vi "enable logging.vi"(6 "call chain index (1)":i32, 7 "vi ref (caller)":refnum<vi>, 8 "error in (no error)":errorcluster, 10 "save pre-launch status (F)":bool, 11 "log file path":path) -> (0 "error out":errorcluster)   [LabVIEW 2024, in "status manager.lvlib"]
uses:
  status manager.lvlib
  <vilib>/Hampel Software Engineering/HSE Logger/LogLevel.ctl
  logger actions.ctl
  <vilib>/Hampel Software Engineering/HSE Logger/Formatter/HSE_v2_Formatter/HSE_v2_Formatter.lvclass
  <vilib>/Hampel Software Engineering/HSE Logger/Handler/FileHandler/FileHandler.lvclass
  <vilib>/Hampel Software Engineering/HSE Logger/hse-logger.lvlib
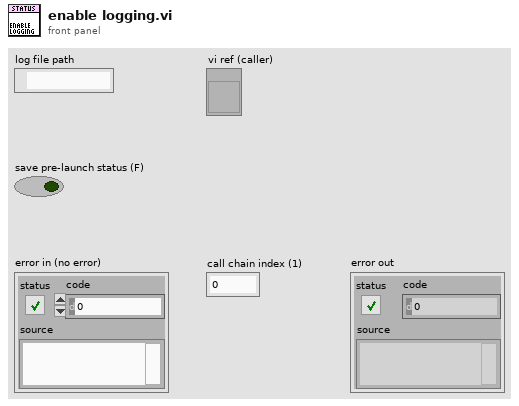
[diagram p1: front panel]
types:
  T1 = typedef "status manager.lvlib/logger actions.ctl" = enum16{"insert", "remove"}
  T2 = typedef "hse-logger.lvlib/LogLevel.ctl" = enum16{"DEBUG", "INFO", "WARNING", "ERROR", "CRITICAL"}
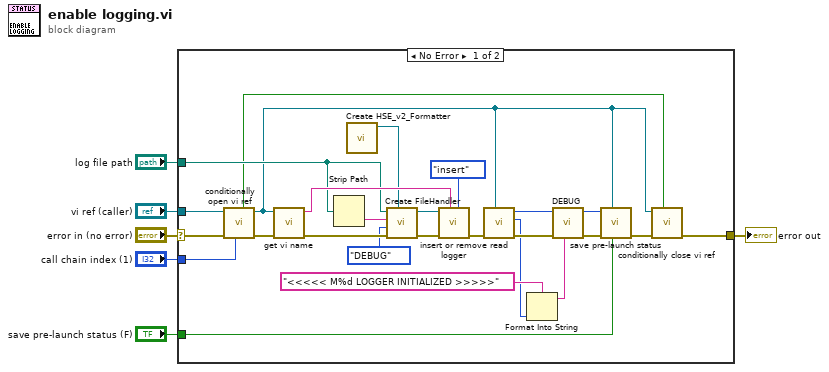
[diagram p0: block diagram]
diagram:
  n1 = case shown="No Error" "error in (no error)" {
    selector: "error in (no error)" -> [w19 w32]
    tunnel: "log file path" -> [w26 _]
    tunnel: "vi ref (caller)" -> [w17 _]
    tunnel: [w22 w32] -> w3
    tunnel: "save pre-launch status (F)" -> [w20 _]
    tunnel: "call chain index (1)" -> [w9 _]
    frame No Error {
      n2 = call "conditionally open vi ref.vi"("call chain index (1)"=w9, "error in (no error)"=w19, "vi ref in"=w17) -> ("error out"=w18:errorcluster, "vi ref out"=w8:refnum<vi>, "new ref?"=w16:bool)  [unwired: 6 in]
      n3 = call "get vi name.vi"("error in (no error)"=w18, "vi ref"=w8) -> ("error out"=w30:errorcluster, "vi name"=w31:string)  [unwired: 8 in]
      n4 = Strip Path(path=w26) -> (name=w25:string)  [unwired: 1 out]
      n5 = call <vilib>:"Create HSE_v2_Formatter.vi"() -> ("HSE_v2_Formatter out"=w27:refnum<class "HSE_v2_Formatter.lvclass">)  [unwired: 10 in, 1 out]
      n6 = call <vilib>:"Create FileHandler.vi"("Formatter.lvclass"=w27, "error in"=w30, "Level"=LogLevel."DEBUG", "Name"=w25, "Filepath"=w26) -> ("error out"=w15:errorcluster, "FileHandler out"=w13:refnum<class "FileHandler.lvclass">)  [unwired: 5 in]
      n7 = call "insert or remove logger.vi"("action"=logger_actions."insert", "handler name"=w31, "error in (no error)"=w15, "handler to insert"=w13) -> ("error out"=w14:errorcluster)  [unwired: 7 in]
      n8 = call "read.vi"("vi ref (caller)"=w8, "error in (no error)"=w14) -> ("error out"=w11:errorcluster, "module id"=w10:i32, "status control id"=w7:i32)  [unwired: 7 in]
      n9 = Format Into String(format string="<<<<< M%d LOGGER INITIALIZED >>>>>", w10) -> (resulting string=w23:string)  [unwired: 2 in, 1 out]
      n10 = call <vilib>:"DEBUG.vi"("Message"=w23, "error in"=w11) -> ("error out"=w29:errorcluster)  [unwired: 9 in]
      n11 = call "save pre-launch status.vi"("save pre-launch status"=w20, "vi ref"=w8, "error in (no error)"=w29, "status control id"=w7) -> ("error out"=w21:errorcluster)  [unwired: 7 in]
      n12 = call "conditionally close vi ref.vi"("new ref?"=w16, "error in (no error)"=w21, "vi ref"=w8) -> ("error out"=w22:errorcluster)  [unwired: 8 in]
    }
    frame Error {
    }
  }
  "error out" <- w3
